vi "Init.vi"(10 "Input":string, 11 "Circular Buffer in":refnum<class "Circular Buffer.lvclass">) -> (3 "Circular Buffer out":refnum<class "Circular Buffer.lvclass">)   [LabVIEW 2021, in "d20.lvlib" / "Circular Buffer.lvclass"]
uses:
  Circular Buffer.lvclass
  INode/INode.lvclass
  Node/Node.lvclass
  Circular Buffer.lvclass/Circular Buffer.ctl
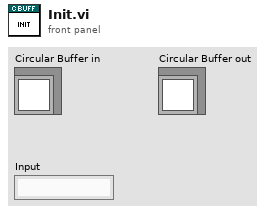
[diagram p1: front panel]
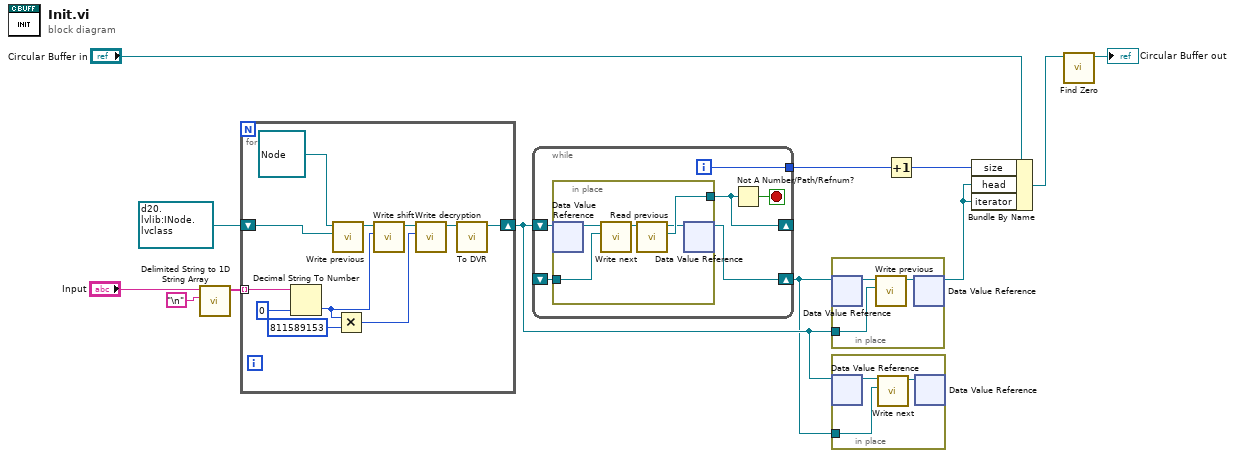
[diagram p0: block diagram]
diagram:
  n1 = call <vilib>:"Delimited String to 1D String Array.vi"("delimiter"="\n", "delimited string"="Input") -> ("string array"=w9:string[])  [unwired: 9 in]
  n2 = for {
    tunnel: w9 -> [w23] mode=indexing
    shift-right: [w21] -> w10
    shift-left: refnum<data-value> refnum ("next") -> [w19]
    n3 = Decimal String To Number(string=w23, default (0L)=i64 0 ("default (0 I32)")) -> (number=w16:i64)  [unwired: 1 in, 1 out]
    n4 = call-dynamic "Write previous.vi"("previous"=w19, "Node in"=refnum<class "Node.lvclass"> refnum ("d20.lvlib:Node.lvclass")) -> ("Node out"=w17:refnum<class "Node.lvclass">)  [unwired: 9 in]
    n5 = Multiply(x=w16, y=i64 811589153) -> (x*y=w14:i64)
    n6 = call "Write shift.vi"("shift"=w16, "Node in"=w17) -> ("Node out"=w15:refnum<class "Node.lvclass">)  [unwired: 9 in]
    n7 = call "Write decryption.vi"("decryption"=w14, "Node in"=w15) -> ("Node out"=w13:refnum<class "Node.lvclass">)  [unwired: 9 in]
    n8 = call-dynamic "To DVR.vi"("Node"=w13) -> ("DVR"=w21:refnum<data-value>)  [unwired: 10 in]
  }
  n9 = while {
    shift-right: [w28] -> w5
    shift-left: _ -> [w24]
    shift-right: [w27] -> _
    shift-left: w10 -> [w29]
    tunnel: [w25] -> w7
    i -> [w25]
    stop <- w26 stop-if-true
    n10 = in-place {
      in-place-border: w24 -> [w34]
      in-place-border: [w32] -> w27
      n11 = in-place-dvr #1(w29) -> (w30:refnum<class "INode.lvclass">)  [unwired: 1 out]
      n12 = call-dynamic "Write next.vi"("next"=w34, "Node in"=w30) -> ("Node out"=w33:refnum<class "INode.lvclass">)  [unwired: 9 in]
      n13 = call-dynamic "Read previous.vi"("Node in"=w33) -> ("previous"=w32:refnum<data-value>, "Node out"=w31:refnum<class "INode.lvclass">)  [unwired: 9 in]
      n14 = in-place-dvr #1(w31) -> (w28:refnum<data-value>)  [unwired: 1 out]
    }
    n15 = Not A Number/Path/Refnum?(number/path/refnum=w27) -> (NaN/Path/Refnum?=w26:bool)
  }
  n16 = in-place {
    in-place-border: w10 -> [w37]
    n17 = in-place-dvr #2(w5) -> (w35:refnum<class "INode.lvclass">)  [unwired: 1 out]
    n18 = call-dynamic "Write previous.vi"("previous"=w37, "Node in"=w35) -> ("Node out"=w36:refnum<class "INode.lvclass">)  [unwired: 9 in]
    n19 = in-place-dvr #2(w36) -> (w4:refnum<data-value>)  [unwired: 1 out]
  }
  n20 = in-place {
    in-place-border: w5 -> [w40]
    n21 = in-place-dvr #3(w10) -> (w38:refnum<class "INode.lvclass">)  [unwired: 1 out]
    n22 = call-dynamic "Write next.vi"("next"=w40, "Node in"=w38) -> ("Node out"=w39:refnum<class "INode.lvclass">)  [unwired: 9 in]
    n23 = in-place-dvr #3(w39) -> ()  [unwired: 2 out]
  }
  n24 = Increment(x=w7) -> (x+1=w6:i32)
  n25 = Bundle By Name(cluster="Circular Buffer in", "size"=w6, "head"=w4, "iterator"=w4) -> (w3:refnum<class "Circular Buffer.lvclass">)
  n26 = call "Find Zero.vi"("Circular Buffer in"=w3) -> ("Circular Buffer out"=→"Circular Buffer out":refnum<class "Circular Buffer.lvclass">)  [unwired: 10 in]
